vi "replaceFileExtension.vi"(10 "newExtension":string, 11 "pathIn":path) -> (1 "original\"Extension\"":string, 3 "pathOut":path)   [LabVIEW 2022 SP3]
panel:
  # "Sick of writing this on the diagram again and again..!  TCRL 2021-06-24"
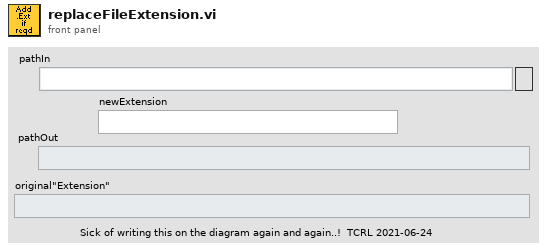
[diagram p1: front panel]
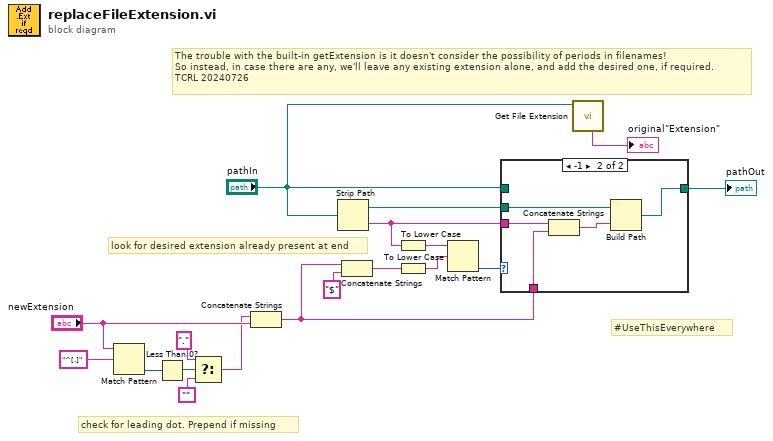
[diagram p0: block diagram]
diagram:
  # "look for desired extension already present at end"
  # "check for leading dot. Prepend if missing"
  # "The trouble with the built-in getExtension is it doesn't consider the possibility of periods in filenames!\nSo instead, in case there are any, we'll leave any existing extension alone, and add the desired one, if required.\nTCRL 20240726"
  # "#UseThisEverywhere"
  n1 = Match Pattern(string="newExtension", regular expression="^[.]") -> (offset past match=w10:i32)  [unwired: 1 in, 3 out]
  n2 = Less Than 0?(x=w10) -> (x < 0?=w9:bool)
  n3 = Select(t=".", s=w9, f="") -> (s? t:f=w5:string)
  n4 = Concatenate Strings(w5, "newExtension") -> (w4:string)
  n5 = Strip Path(path="pathIn") -> (stripped path=w17:path, name=w14:string)
  n6 = Concatenate Strings(w4, "$" ("string")) -> (w3:string)
  n7 = To Lower Case(string=w14) -> (all lower case string=w16:string)
  n8 = To Lower Case(string=w3) -> (all lower case string=w2:string)
  n9 = Match Pattern(string=w16, regular expression=w2) -> (offset past match=w13:i32)  [unwired: 1 in, 3 out]
  n10 = case shown="-1" w13 {
    tunnel: [w19 w24] -> w18
    tunnel: w17 -> [_ w23]
    tunnel: w14 -> [_ w21]
    tunnel: w4 -> [_ w20]
    tunnel: "pathIn" -> [w19 _]
    frame 0, Default {
    }
    frame -1 {
      n11 = Concatenate Strings(w21, w20) -> (w22:string)
      n12 = Build Path(base path=w23, name or relative path=w22) -> (appended path=w24:path)
    }
  }
  "pathOut" <- w18
  n13 = call <vilib>:"Get File Extension.vi"("file"="pathIn") -> ("unmodified file extension"=→"original\"Extension\"":string)  [unwired: 6 in, 4 out]
